vi "TestExec.Append Fault Code Prefix.vi"(7 "Positive(F)\\Negative(T)":bool, 9 "FaultCode":i32, 10 "FaultCode Prefix":i32) -> (1 "New Fault Code":i32)   [LabVIEW 2018]
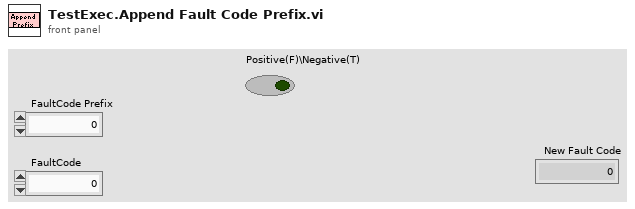
[diagram p1: front panel]
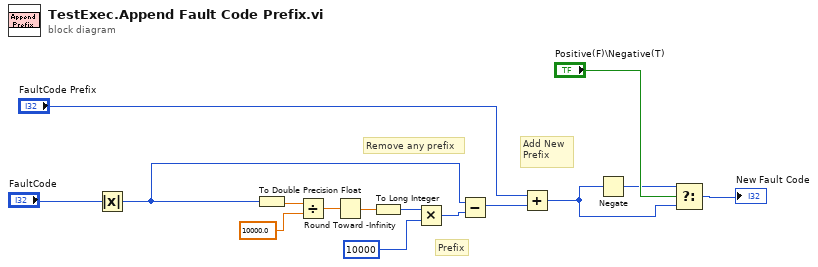
[diagram p0: block diagram]
diagram:
  # "Add New\nPrefix"
  # "Remove any prefix"
  # "Prefix"
  n1 = Absolute Value(x="FaultCode") -> (abs(x)=w3:i32)
  n2 = To Double Precision Float(number=w3) -> (double precision float=w15:dbl)
  n3 = Divide(x=w15, y=10000.0) -> (x/y=w13:dbl)
  n4 = Round Toward -Infinity(1:w13) -> (0:w12:dbl)
  n5 = To Long Integer(number=w12) -> (32bit integer=w11:i32)
  n6 = Multiply(x=w11, y=10000) -> (x*y=w9:i32)
  n7 = Subtract(x=w3, y=w9) -> (x-y=w8:i32)
  n8 = Add(x="FaultCode Prefix", y=w8) -> (x+y=w2:i32)
  n9 = Negate(x=w2) -> (-x=w5:i32)
  n10 = Select(t=w5, s="Positive(F)\\Negative(T)", f=w2) -> (s? t:f=→"New Fault Code":i32)
